vi "Make filepath.vi"(8 "error in (no error)":errorcluster, 9 "is cxd file path?":bool, 10 "base path":path, 11 "DAQOrcaFlash in":refnum<class "DAQOrcaFlash.lvclass">) -> (0 "error out":errorcluster, 2 "filepath out":path, 3 "DAQOrcaFlash out":refnum<class "DAQOrcaFlash.lvclass">)   [LabVIEW 2012, in "DAQOrcaFlash.lvclass"]
uses:
  DAQOrcaFlash.lvclass
  DAQOrcaFlash.lvclass/DAQOrcaFlash.ctl
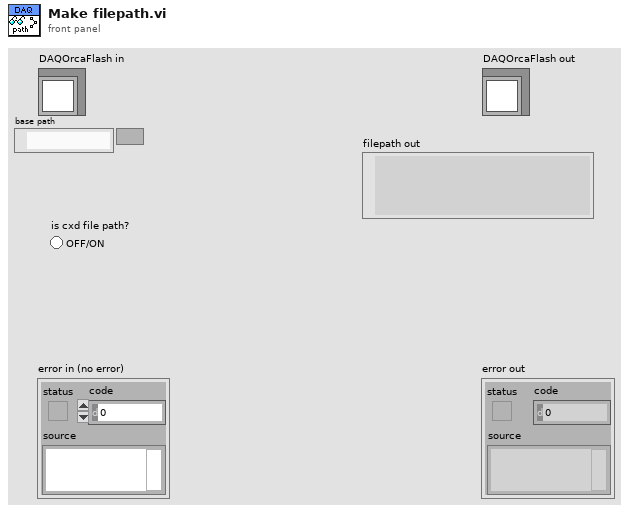
[diagram p1: front panel]
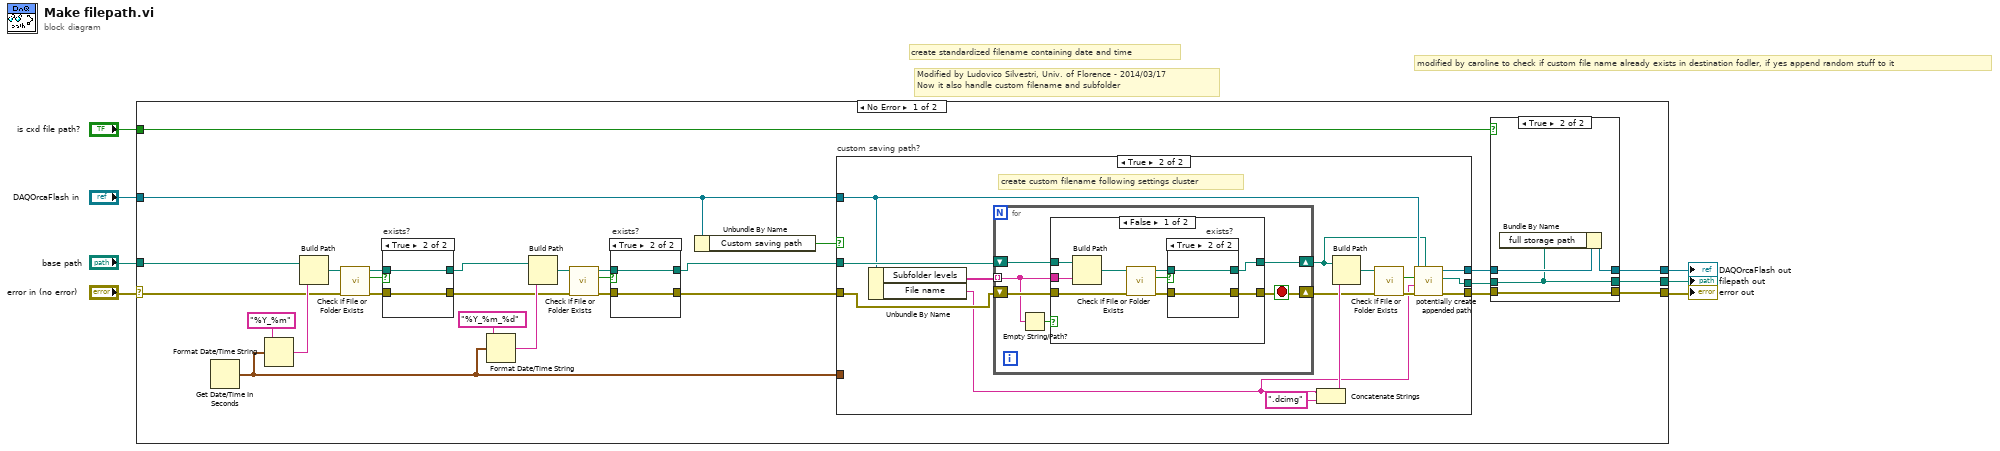
[diagram p0: block diagram]
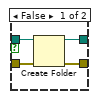
[diagram p3: hidden frame]
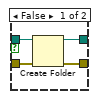
[diagram p4: hidden frame]
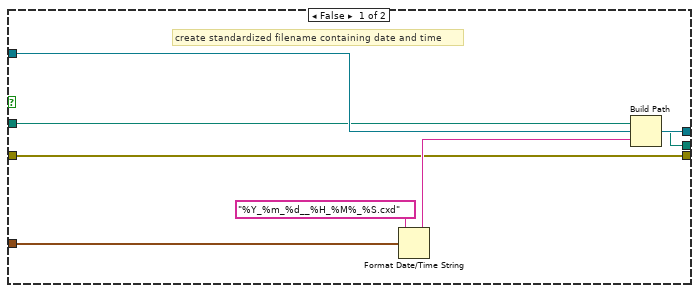
[diagram p5: hidden frame]
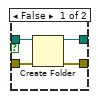
[diagram p6: hidden frame]
diagram:
  # "modified by caroline to check if custom file name already exists in destination fodler, if yes append random stuff to it"
  # "create standardized filename containing date and time"
  # "Modified by Ludovico Silvestri, Univ. of Florence - 2014/03/17\nNow it also handle custom filename and subfolder"
  n1 = case shown="No Error" "error in (no error)" {
    selector: "error in (no error)" -> [w20 w101]
    tunnel: [w10 w101] -> w6
    tunnel: [w9 w100] -> w5
    tunnel: "DAQOrcaFlash in" -> [w19 w100]
    tunnel: "base path" -> [w15 _]
    tunnel: "is cxd file path?" -> [w11 _]
    tunnel: [w8 _] -> w1
    frame No Error {
      n2 = Get Date/Time In Seconds() -> (seconds since 1Jan1904=w17:timestamp)
      n3 = Format Date/Time String(time format string (%c)="%Y_%m", seconds (now)=w17) -> (date/time string=w34:string)  [unwired: 1 in]
      n4 = Build Path(base path=w15, name or relative path=w34) -> (appended path=w32:path)
      n5 = call <vilib>:"Check if File or Folder Exists.vi"("error in (no error)"=w20, "path"=w32) -> ("error out"=w29:errorcluster, "file or folder exists?"=w31:bool, "dup path"=w30:path)  [unwired: 7 in]
      n6 = case "exists?" shown="True" w31 {
        tunnel: w30 -> [w51 w53]
        tunnel: w29 -> [w52 w54]
        tunnel: [w50 w53] -> w21
        tunnel: [w49 w54] -> w22
        frame False {
          n7 = Create Folder(path (use dialog)=w51, error in=w52) -> (created path=w50:path, error out=w49:errorcluster)  [unwired: 1 in, 1 out]
        }
        frame True {
        }
      }
      n8 = Format Date/Time String(time format string (%c)="%Y_%m_%d", seconds (now)=w17) -> (date/time string=w24:string)  [unwired: 1 in]
      n9 = Build Path(base path=w21, name or relative path=w24) -> (appended path=w28:path)
      n10 = call <vilib>:"Check if File or Folder Exists.vi"("error in (no error)"=w22, "path"=w28) -> ("error out"=w25:errorcluster, "file or folder exists?"=w27:bool, "dup path"=w26:path)  [unwired: 7 in]
      n11 = case "exists?" shown="True" w27 {
        tunnel: w26 -> [w45 w47]
        tunnel: w25 -> [w46 w48]
        tunnel: [w44 w47] -> w16
        tunnel: [w43 w48] -> w18
        frame False {
          n12 = Create Folder(path (use dialog)=w45, error in=w46) -> (created path=w44:path, error out=w43:errorcluster)  [unwired: 1 in, 1 out]
        }
        frame True {
        }
      }
      n13 = Unbundle By Name(w19) -> ("Custom saving path"=w35:bool)
      n14 = case "custom saving path?" shown="True" w35 {
        tunnel: w18 -> [w57 w75]
        tunnel: w19 -> [w60 w69]
        tunnel: [w57 w71] -> w12
        tunnel: [w59 w62] -> w13
        tunnel: [w60 w70] -> w14
        tunnel: w17 -> [w56 _]
        tunnel: w16 -> [w55 w72]
        frame False {
          # "create standardized filename containing date and time"
          n15 = Format Date/Time String(time format string (%c)="%Y_%m_%d__%H_%M%_%S.cxd", seconds (now)=w56) -> (date/time string=w61:string)  [unwired: 1 in]
          n16 = Build Path(base path=w55, name or relative path=w61) -> (appended path=w59:path)
        }
        frame True {
          # "create custom filename following settings cluster"
          n17 = Unbundle By Name(w69) -> ("Subfolder levels"=w76:string[], "File name"=w64:string)
          n18 = for {
            tunnel: w76 -> [w78] mode=indexing
            shift-right: [w80] -> w63
            shift-left: w72 -> [w82]
            shift-right: [w79] -> w68
            shift-left: w75 -> [w81]
            stop <- w79 stop-if-true
            n19 = Empty String/Path?(string/path=w78) -> (empty?=w77:bool)
            n20 = case shown="False" w77 {
              tunnel: w82 -> [w91 w98]
              tunnel: w78 -> [w90 _]
              tunnel: w81 -> [w85 w99]
              tunnel: [w84 w98] -> w80
              tunnel: [w83 w99] -> w79
              frame False {
                n21 = Build Path(base path=w91, name or relative path=w90) -> (appended path=w86:path)
                n22 = call <vilib>:"Check if File or Folder Exists.vi"("error in (no error)"=w85, "path"=w86) -> ("error out"=w89:errorcluster, "file or folder exists?"=w87:bool, "dup path"=w88:path)  [unwired: 7 in]
                n23 = case "exists?" shown="True" w87 {
                  tunnel: w88 -> [w94 w96]
                  tunnel: w89 -> [w95 w97]
                  tunnel: [w93 w96] -> w84
                  tunnel: [w92 w97] -> w83
                  frame False {
                    n24 = Create Folder(path (use dialog)=w94, error in=w95) -> (created path=w93:path, error out=w92:errorcluster)  [unwired: 1 in, 1 out]
                  }
                  frame True {
                  }
                }
              }
              frame True {
              }
            }
          }
          n25 = Concatenate Strings(w64, ".dcimg" ("string")) -> (w73:string)
          n26 = Build Path(base path=w63, name or relative path=w73) -> (appended path=w66:path)
          n27 = call <vilib>:"Check if File or Folder Exists.vi"("error in (no error)"=w68, "path"=w66) -> ("error out"=w67:errorcluster, "file or folder exists?"=w65:bool)  [unwired: 7 in, 1 out]
          n28 = call-dynamic "potentially create appended path.vi"("base path"=w63, "error in (no error)"=w67, "File name"=w64, "Boolean"=w65, "DAQOrcaFlash in"=w69) -> ("error out"=w71:errorcluster, "file path"=w62:path, "DAQOrcaFlash out"=w70:refnum<class "DAQOrcaFlash.lvclass">)  [unwired: 4 in]
        }
      }
      n29 = case shown="True" w11 {
        tunnel: w14 -> [w38 w42]
        tunnel: [w38 w41] -> w9
        tunnel: w13 -> [w37 w40]
        tunnel: [w37 w40] -> w8
        tunnel: w12 -> [w36 w39]
        tunnel: [w36 w39] -> w10
        frame False {
        }
        frame True {
          n30 = Bundle By Name(cluster=w42, "full storage path"=w40) -> (w41:refnum<class "DAQOrcaFlash.lvclass">)
        }
      }
    }
    frame Error {
    }
  }
  "error out" <- w6
  "DAQOrcaFlash out" <- w5
  "filepath out" <- w1
